vi "Write Instrument Descriptor.vi"(8 "error in (no error)":errorcluster, 10 "Instrument Descriptor":refnum<k15>="Dev1", 11 "NI DMM in":refnum<class "NI DMM.lvclass">) -> (0 "error out":errorcluster, 3 "NI DMM out":refnum<class "NI DMM.lvclass">)   [LabVIEW 2020, in "NI DMM.lvclass"]
uses:
  NI DMM.lvclass
  NI DMM.lvclass/NI DMM.ctl
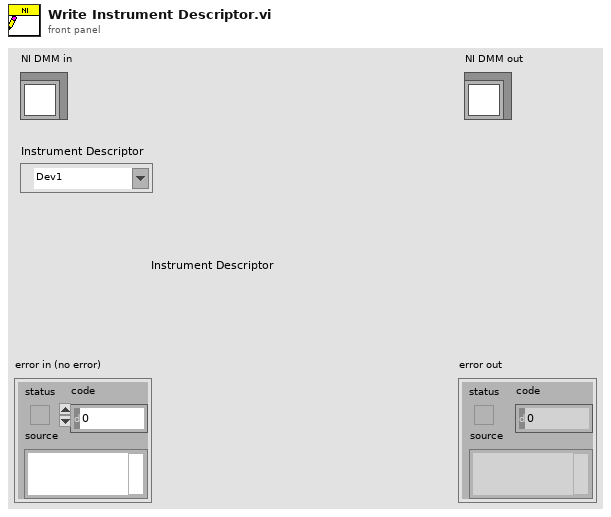
[diagram p1: front panel]
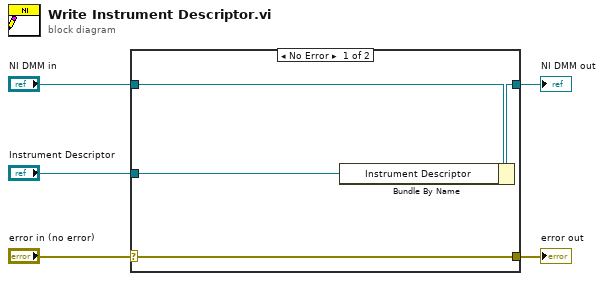
[diagram p0: block diagram]
diagram:
  n1 = case shown="No Error" "error in (no error)" {
    selector: "error in (no error)" -> [w9 w10]
    tunnel: [w9 w10] -> w4
    tunnel: [w7 w11] -> w2
    tunnel: "NI DMM in" -> [w8 w11]
    tunnel: "Instrument Descriptor" -> [w6 _]
    frame No Error {
      n2 = Bundle By Name(cluster=w8, "Instrument Descriptor"=w6) -> (w7:refnum<class "NI DMM.lvclass">)
    }
    frame Error {
    }
  }
  "error out" <- w4
  "NI DMM out" <- w2
